vi "MB Verbindung herstellen.vi"(8 "error in (no error)":errorcluster caption="Fehler (Eingang, kein Fehler)", 11 "Steuerung PNS Eingang":refnum<class "Steuerung PNS.lvclass">) -> (0 "error out":errorcluster caption="Fehler (Ausgang)", 3 "Steuerung PNS Ausgang":refnum<class "Steuerung PNS.lvclass">)   [LabVIEW 2020, in "Steuerung PNS.lvclass"]
doc: "Low Level Modbus Kommunikation mit Timeouts mit der IP Adresse aus dem Objekt (wieder) herstellen.\nWichtig: die Modebus Referenz (TCP master instance) wird im Objekt gespeichert, und die neue Objektreferenz muss von nun an verwendet werden, um kommunizieren zu können. \nRIW"
uses:
  Steuerung PNS.lvclass
  Steuerung PNS.lvclass/Steuerung PNS.ctl
  <vilib>/NI/Modbus Library/API/Modbus API.lvclass/Modbus API.ctl
  <vilib>/NI/Modbus Library/Transmission Data Unit/Transmission Data Unit.lvclass/Transmission Data Unit.ctl
  <vilib>/NI/Modbus Library/Transmission Data Unit/Write Unit ID.vi
  <vilib>/NI/Modbus Library/API/Read Transmission Data Unit.vi
  <vilib>/NI/Modbus Library/API/Write Transmission Data Unit.vi
  <vilib>/NI/Modbus Library/API/Master/Modbus Master.lvclass
  C:/Program Files (x86)/National Instruments/LabVIEW 2020/vi.lib/NI/Modbus Library/API/Modbus API.lvclass
  <vilib>/NI/Modbus Library/API/Wrapper/Create TCP Master.vi
  <vilib>/NI/Modbus Library/API/Wrapper/API Main.lvlib
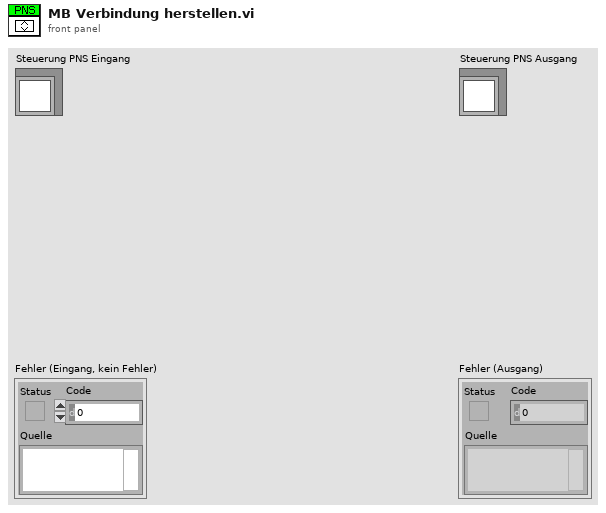
[diagram p1: front panel]
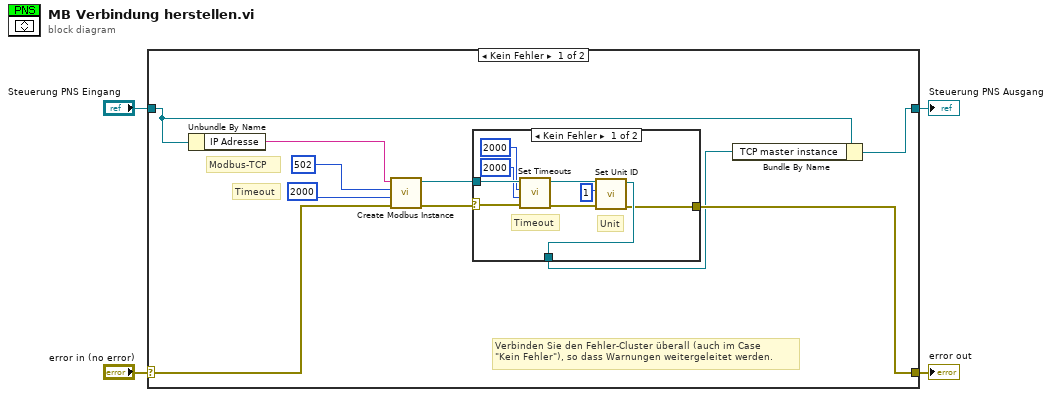
[diagram p0: block diagram]
diagram:
  n1 = case shown="Kein Fehler" "error in (no error)" {
    selector: "error in (no error)" -> [w9 w27]
    tunnel: [w8 w27] -> w3
    tunnel: [w5 w26] -> w1
    tunnel: "Steuerung PNS Eingang" -> [w6 w26]
    frame No Error {
      # "Timeout"
      # "Modbus-TCP"
      # "Verbinden Sie den Fehler-Cluster überall (auch im Case\n\"Kein Fehler\"), so dass Warnungen weitergeleitet werden."
      n2 = Unbundle By Name(w6) -> ("IP Adresse"=w10:string)
      n3 = call-poly <vilib>:"Create Modbus Instance.vi"("error in"=w9, "connect timeout ms"=2000 ("Timeout in ms (60000)"), "port (502)"=u16 502 ("Netzwerk-Port oder -Dienst"), "address"=w10) -> ("error out"=w12:errorcluster, "TCP master instance"=w11:refnum<class "Modbus Master.lvclass">)  [unwired: 6 in]
      n4 = case shown="Kein Fehler" w12 {
        selector: w12 -> [w18 w24]
        tunnel: w11 -> [w23 w25]
        tunnel: [w21 w25] -> w7
        tunnel: [w15 w24] -> w8
        frame No Error {
          # "Unit"
          # "Timeout"
          n5 = call <vilib>:"Set Timeouts.vi"("error in"=w18, "write operation timeout"=2000, "read operation timeout"=2000, "Modbus master in"=w23) -> ("error out"=w19:errorcluster, "Modbus master out"=w22:refnum<class "Modbus Master.lvclass">)  [unwired: 6 in]
          n6 = call <vilib>:"Set Unit ID.vi"("error in"=w19, "unit ID"=u8 1, "Modbus master in"=w22) -> ("error out"=w15:errorcluster, "Modbus master out"=w21:refnum<class "Modbus Master.lvclass">)  [unwired: 7 in]
        }
        frame Error {
        }
      }
      n7 = Bundle By Name(cluster=w6, "TCP master instance"=w7) -> (w5:refnum<class "Steuerung PNS.lvclass">)
    }
    frame Error {
    }
  }
  "error out" <- w3
  "Steuerung PNS Ausgang" <- w1
